vi "Banda_HMI_Test_Bidir.vi"() -> ()   [LabVIEW 2026]
uses:
  <vilib>/Modbus/master/Create Master Instance (Serial).vi
  <vilib>/Modbus/master/Modbus Master.lvclass
panel:
  in  "stop":bool
  out "Sobrecalentamiento":bool
  out "Contador de piezas":dbl
  out "Temperatura":dbl(slide) scale=0.0..100.0
  out "Sensor de Presencia":bool
  in  "Brazo clasificador":bool
  in  "Velocidad Motor":dbl(knob) scale=0.0..100.0
  in  "Motor ON/OFF":bool
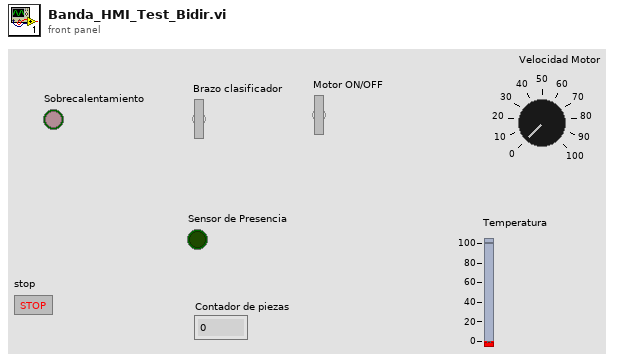
[diagram p1: front panel]
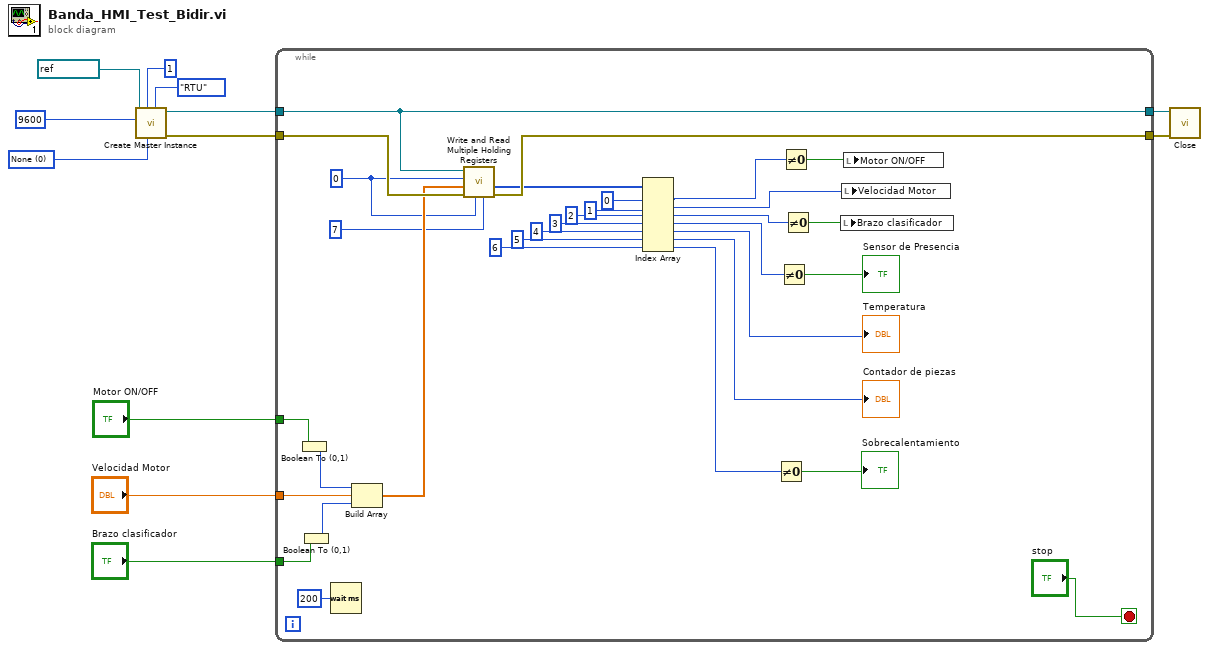
[diagram p0: block diagram]
diagram:
  w9 = u16 0 items=["None", "Odd", "Even"] ("parity (Even)")
  n1 = call-poly <vilib>:"Create Master Instance.vi"("serial type"=enum16{"RTU", "ASCII"}."RTU", "parity (Even)"=w9, "unit ID"=u8 1, "baud rate (9600)"=u32 9600, "VISA resource name"=refnum<visa-resource-name> "COM1") -> ("error out"=w6:errorcluster, "serial master instance"=w5:refnum<class "Modbus Master.lvclass">)  [unwired: 5 in]
  n2 = while {
    tunnel: w5 -> [w35]
    tunnel: [w35] -> w12
    tunnel: w6 -> [w34]
    tunnel: [w33] -> w4
    tunnel: "Motor ON/OFF" -> [w20]
    tunnel: "Velocidad Motor" -> [w16]
    tunnel: "Brazo clasificador" -> [w19]
    stop <- "stop" stop-if-true
    w14 = u16 0 ("starting address")
    n3 = Boolean To (0,1)(Boolean=w20) -> (0, 1=w18:i16)
    n4 = Boolean To (0,1)(Boolean=w19) -> (0, 1=w17:i16)
    n5 = Wait (ms)(milliseconds to wait=u32 200) -> ()  [unwired: 1 out]
    n6 = Build Array(w18, w16, w17) -> (w15:dbl[])
    n7 = call-dynamic "Write and Read Multiple Holding Registers.vi"("read count"=u16 7 ("number of holding registers"), "read operation starting address"=w14, "error in (no error)"=w34, "values to write"=w15, "write operation starting address"=w14, "Modbus master in"=w35) -> ("error out"=w33:errorcluster, "values read"=w32:u16[])  [unwired: 3 in, 1 out]
    n8 = Index Array(array=w32, index #1=0 ("index"), index #2=1 ("index"), index #3=2 ("index"), index #4=3 ("index"), index #5=4 ("index"), index #6=5 ("index"), index #7=6 ("index")) -> (element #1=w21:u16, element #2=w23:u16, element #3=w24:u16, element #4=w26:u16, element #5=→"Temperatura":u16, element #6=→"Contador de piezas":u16, element #7=w30:u16)
    n9 = Not Equal To 0?(x=w30) -> (x != 0?=→"Sobrecalentamiento":bool)
    n10 = Not Equal To 0?(x=w26) -> (x != 0?=→"Sensor de Presencia":bool)
    n11 = Not Equal To 0?(x=w21) -> (x != 0?=w22:bool)
    n12 = Not Equal To 0?(x=w24) -> (x != 0?=w25:bool)
    n13 = local write "Brazo clasificador"(w25) -> ()
    n14 = local write "Velocidad Motor"(w23) -> ()
    n15 = local write "Motor ON/OFF"(w22) -> ()
  }
  n16 = call-dynamic "Close.vi"("error in (no error)"=w4, "Modbus master in"=w12) -> ()  [unwired: 9 in, 1 out]
